vi "show2.vi"(6 "lines":i32, 7 "x":i32, 8 "reference":refnum<vi>, 9 "OPTION":string="i", 10 "first letter to find":string="i", 11 "Array":string[](array[string])=["F", "a", "b", "i", "o"]) -> ()   [LabVIEW 2014]
uses:
  <vilib>/Utility/miscctls.llb/LVRowAndColumnUnsignedTypeDef.ctl
  <vilib>/Utility/miscctls.llb/LVRowAndColumnTypeDef.ctl
  <vilib>/Utility/miscctls.llb/LVBoundsTypeDef.ctl
panel:
  out "output cluster":cluster{i32, i32}
  out "Second":string
  out "First":string
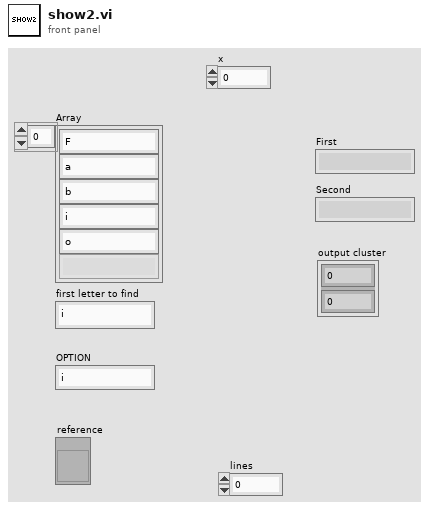
[diagram p1: front panel]
types:
  T1 = typedef "LVRowAndColumnUnsignedTypeDef.ctl" = cluster{"Row":u32, "Column":u32}
  T2 = typedef "LVBoundsTypeDef.ctl" = cluster{"Width":u32, "Height":u32}
  T3 = typedef "LVRowAndColumnTypeDef.ctl" = cluster{"Row":i32, "Column":i32}
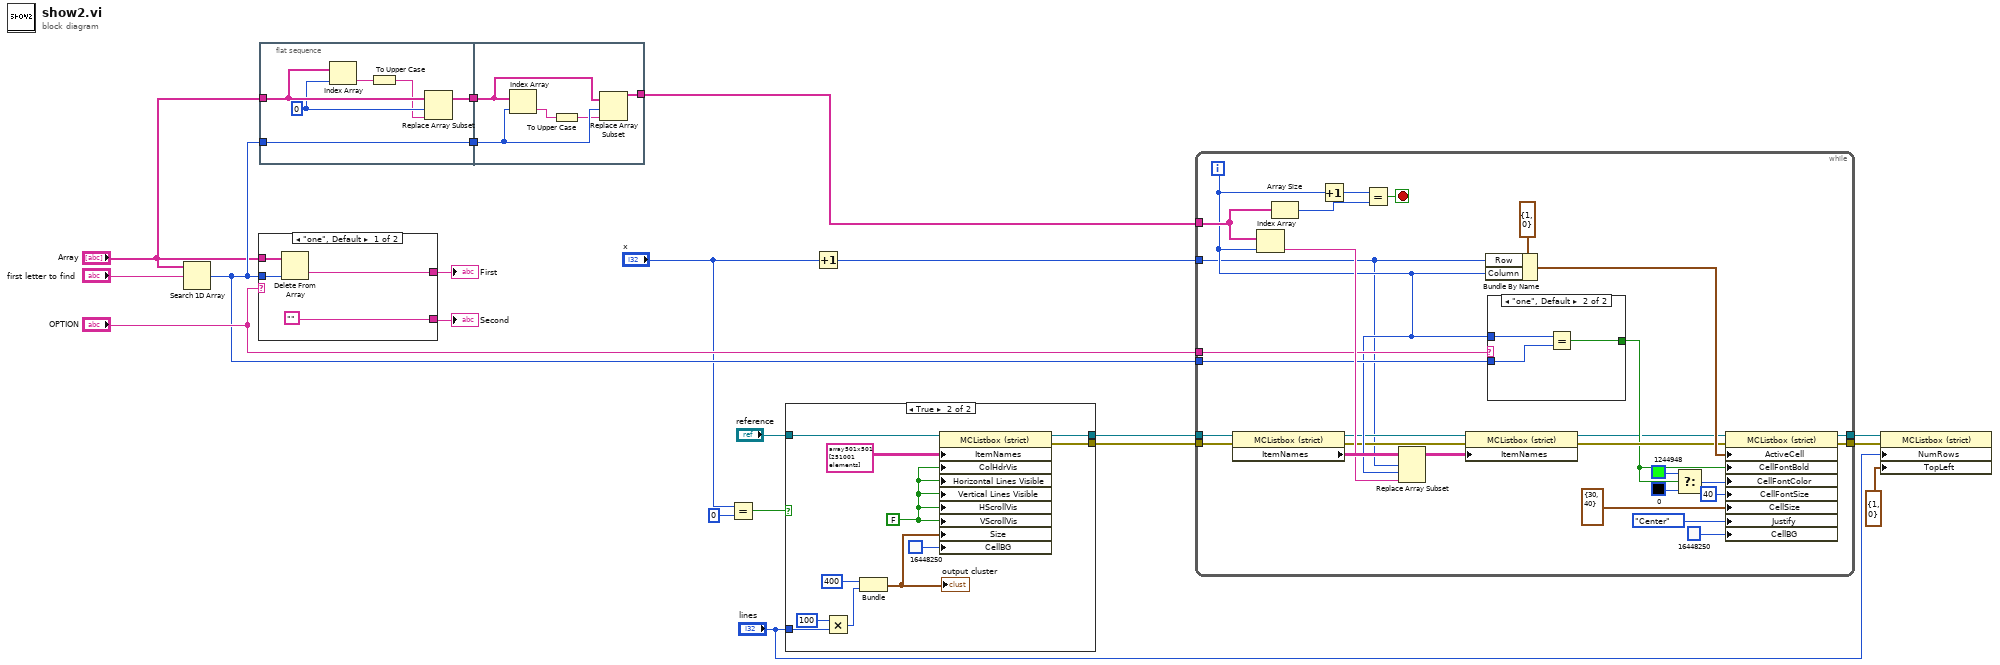
[diagram p0: block diagram]
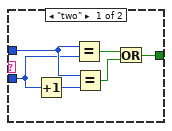
[diagram p3: hidden frame]
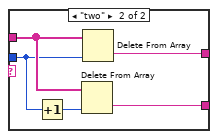
[diagram p4: hidden frame]
diagram:
  n1 = Search 1D Array(1D array="Array", element="first letter to find") -> (index of element=w11:i32)  [unwired: 1 in]
  n2 = case shown="\"one\", Default" "OPTION" {
    tunnel: "Array" -> [w24 w28]
    tunnel: w11 -> [w22 w25]
    tunnel: [w23 w26] -> w19
    tunnel: ["" w27] -> w20
    frame "one", Default {
      n3 = Delete From Array(array=w24, index=w22) -> (deleted portion=w23:string)  [unwired: 1 in, 1 out]
    }
    frame "two" {
      n4 = Increment(x=w25) -> (x+1=w29:i32)
      n5 = Delete From Array(array=w28, index=w29) -> (deleted portion=w27:string)  [unwired: 1 in, 1 out]
      n6 = Delete From Array(array=w28, index=w25) -> (deleted portion=w26:string)  [unwired: 1 in, 1 out]
    }
  }
  "First" <- w19
  "Second" <- w20
  n7 = flat-sequence {
    tunnel: "Array" -> [w35]
    tunnel: [w30] -> w13
    tunnel: [w31] -> w12
    tunnel: w11 -> [w31]
    tunnel: w13 -> [w40]
    tunnel: w12 -> [w39]
    tunnel: [w36] -> w10
    frame #0 {
      w34 = 0 ("index")
      n8 = Index Array(array=w35, index=w34) -> (element=w33:string)
      n9 = To Upper Case(1:w33) -> (0:w32:string)
      n10 = Replace Array Subset(array=w35, new element=w32, index=w34) -> (w30:string[])
    }
    frame #1 {
      n11 = Index Array(array=w40, index=w39) -> (element=w38:string)
      n12 = To Upper Case(1:w38) -> (0:w37:string)
      n13 = Replace Array Subset(array=w40, new element=w37, index=w39) -> (w36:string[])
    }
  }
  n14 = Equal?(x="x", y=0) -> (x = y?=w9:bool)
  n15 = case shown="True" w9 {
    tunnel: [_ w51] -> w17
    tunnel: "reference" -> [w41 w50]
    tunnel: [w41 w49] -> w15
    tunnel: "lines" -> [_ w47]
    frame False {
    }
    frame True {
      w42 = FALSE
      n16 = Multiply(x=100, y=w47) -> (x*y=w44:i32)
      n17 = Bundle(400, w44) -> (w45:cluster{i32, i32})  [unwired: 1 in]
      "output cluster" <- w45
      n18 = property on="Property Node" class="MCListbox (strict)"(reference=w50, "ItemNames"=string[][] array501x501[251001 elements], "ColHdrVis"=w42, "Horizontal Lines Visible"=w42, "Vertical Lines Visible"=w42, "HScrollVis"=w42, "VScrollVis"=w42, "Size"=w45, "CellBG"=u32 16448250) -> (reference out=w49:refnum<vi>, error out=w51:errorcluster)  [unwired: 1 in]
    }
  }
  n19 = Increment(x="x") -> (x+1=w6:i32)
  n20 = while {
    tunnel: w10 -> [w71]
    tunnel: w17 -> [w65]
    tunnel: "OPTION" -> [w76]
    tunnel: w11 -> [w75]
    tunnel: [w66] -> w5
    tunnel: w15 -> [w55]
    tunnel: w6 -> [w54]
    tunnel: [w53] -> w4
    i -> [w70]
    stop <- w68 stop-if-true
    n21 = property on="Property Node" class="MCListbox (strict)"(reference=w55, error in=w65) -> (reference out=w56:refnum<vi>, error out=w64:errorcluster, "ItemNames"=w81:string[][])
    n22 = Index Array(array=w71, index=w70) -> (element=w80:string)
    n23 = Array Size(array=w71) -> (size(s)=w69:i32)
    n24 = Increment(x=w70) -> (x+1=w67:i32)
    n25 = Equal?(x=w67, y=w69) -> (x = y?=w68:bool)
    n26 = Replace Array Subset(array=w81, new element=w80, index (row)=w54, index (col)=w70) -> (w79:string[][])
    n27 = property on="Property Node" class="MCListbox (strict)"(reference=w56, error in=w64, "ItemNames"=w79) -> (reference out=w57:refnum<vi>, error out=w63:errorcluster)
    n28 = Bundle By Name(cluster=T3 {"Row"=1, "Column"=0} ("Active Cell:Active Cell"), "Row"=w54, "Column"=w70) -> (w77:T3)
    n29 = case shown="\"one\", Default" w76 {
      tunnel: w75 -> [w83 w90]
      tunnel: w70 -> [w85 w89]
      tunnel: [w82 w88] -> w61
      frame "two" {
        n30 = Increment(x=w83) -> (x+1=w84:i32)
        n31 = Equal?(x=w85, y=w83) -> (x = y?=w87:bool)
        n32 = Equal?(x=w85, y=w84) -> (x = y?=w86:bool)
        n33 = Or(x=w87, y=w86) -> (x .or. y?=w82:bool)
      }
      frame "one", Default {
        n34 = Equal?(x=w89, y=w90) -> (x = y?=w88:bool)
      }
    }
    n35 = Select(t=u32 1244948, s=w61, f=u32 0) -> (s? t:f=w60:u32)
    n36 = property on="Property Node" class="MCListbox (strict)"(reference=w57, error in=w63, "ActiveCell"=w77, "CellFontBold"=w61, "CellFontColor"=w60, "CellFontSize"=u32 40 ("Active Cell:Cell Font:Size"), "CellSize"=T2 {"Width"=30, "Height"=40} ("Active Cell:Cell Size"), "Justify"=enum16{"Left", "Center", "Right"}."Center" ("Active Cell:Cell Justification"), "CellBG"=u32 16448250) -> (reference out=w53:refnum<vi>, error out=w66:errorcluster)
  }
  n37 = property on="Property Node" class="MCListbox (strict)"(reference=w4, error in=w5, "NumRows"="lines", "TopLeft"=T1 {"Row"=1, "Column"=0} ("Top Left Visible Cell")) -> ()  [unwired: 2 out]
